vi "CRYCurve Library Socket.vi"(10 "sDataIn":string, 11 "sAction":string) -> (3 "sDataOut":string)   [LabVIEW 2013]
uses:
  Control/CRYCurve Library Cluster.ctl
  CRYSystem/Typedef Control/CRYData Cluster Array.ctl
  CRYSystem/Typedef Control/CRYData Cluster.ctl
  CRYSystem/Typedef Control/CRYResult Cluster Array.ctl
  CRYSystem/Typedef Control/CRYResult Cluster.ctl
  CRYSystem/Typedef Control/CRYWaveform Cluster Array.ctl
  CRYSystem/Typedef Control/CRYWaveform Cluster.ctl
  Global/CRYCurve Library Global.vi
  CRYProject/CRYProject Editor Global.vi
panel:
  in  "CurLib Cluster":T1 {"Waveforms"."Y dB ref" format="%.1f"; "Waveforms"."Y axis" items=["Log", "Lin"]; "Waveforms"."Y data" items=["dB", "Lin"]; "Waveforms"."X data" items=["dB", "Lin"]; "Values"."Z data" items=["dB", "Lin"]; "Values"."X data" items=["dB", "Lin"]; "Values"."Y data" items=["dB", "Lin"]; "Values"."Z dB ref" format="%.1f"; "Values"."Z axis" items=["Log", "Lin"]; "Values"."X dB ref" format="%.1f"; "Values"."X axis" items=["Log", "Lin"]; "Values"."Y axis" items=["Log", "Lin"]; "Values"."Y dB ref" format="%.1f"; "Values"."Curve"."z" format="%.2f"; "Values"."Curve"."y" format="%.2f"; "Values"."Curve"."x" format="%.2f"; "Results"."Margin" format="%.2f"; "Curves"."Z data" items=["dB", "Lin"]; "Curves"."X data" items=["dB", "Lin"]; "Curves"."Y data" items=["dB", "Lin"]; "Curves"."Z dB ref" format="%.1f"; "Curves"."Z axis" items=["Log", "Lin"]; "Curves"."X dB ref" format="%.1f"; "Curves"."X axis" items=["Log", "Lin"]; "Curves"."Y axis" items=["Log", "Lin"]; "Curves"."Y dB ref" format="%.1f"; "Curves"."Curve"."z" format="%.2f"; "Curves"."Curve"."y" format="%.2f"; "Curves"."Curve"."x" format="%.2f"}
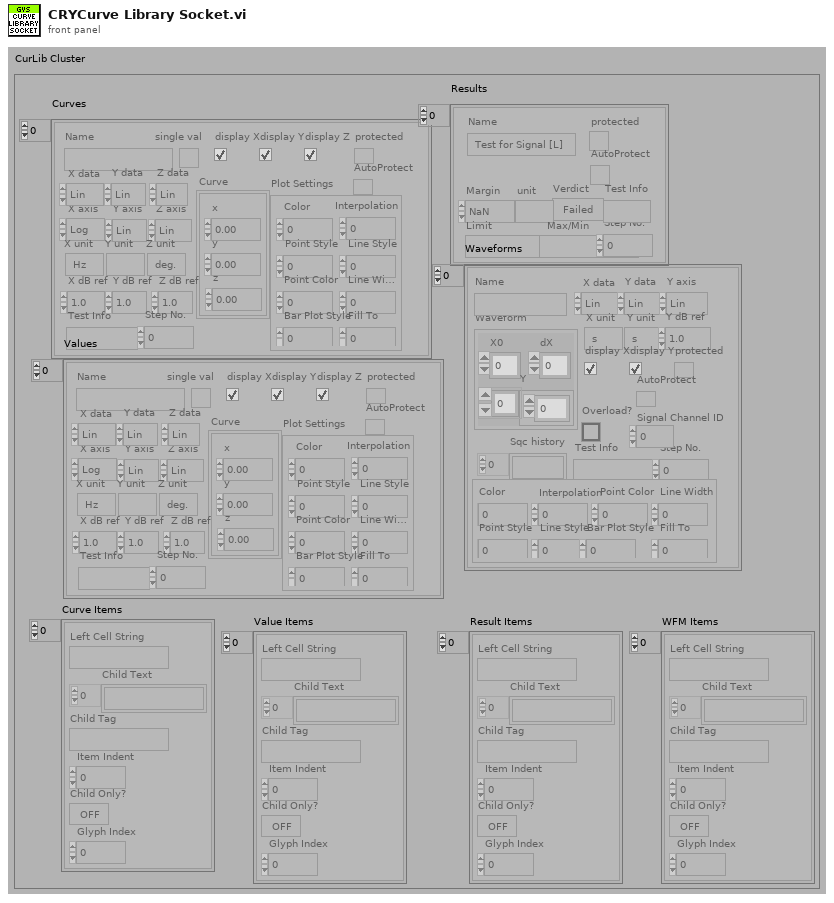
[diagram p1: front panel]
types:
  T1 = typedef "CRYCurve Library Cluster.ctl" = cluster{"Curves":T2, "Results":T4, "Values":T2, "Waveforms":T6, "Curve Items":cluster{"Left Cell String":string, "Child Text":string[], "Child Tag":string, "Item Indent":i32, "Child Only?":bool, "Glyph Index":i32}[], "Value Items":cluster{"Left Cell String":string, "Child Text":string[], "Child Tag":string, "Item Indent":i32, "Child Only?":bool, "Glyph Index":i32}[], "Result Items":cluster{"Left Cell String":string, "Child Text":string[], "Child Tag":string, "Item Indent":i32, "Child Only?":bool, "Glyph Index":i32}[], "WFM Items":cluster{"Left Cell String":string, "Child Text":string[], "Child Tag":string, "Item Indent":i32, "Child Only?":bool, "Glyph Index":i32}[]}
  T2 = typedef "CRYData Cluster Array.ctl" = T3[]
  T3 = typedef "CRYData Cluster.ctl" = cluster{"Name":string, "Curve":cluster{"x":dbl, "y":dbl, "z":dbl}[], "X data":u16, "Y data":u16, "Z data":u16, "X axis":u16, "Y axis":u16, "Z axis":u16, "X unit":string, "Y unit":string, "Z unit":string, "X dB ref":dbl, "Y dB ref":dbl, "Z dB ref":dbl, "single val":bool, "protected":bool, "display X":bool, "display Y":bool, "display Z":bool, "Test Info":string, "Step No.":i32, "Plot Settings":cluster{"Color":u32, "Interpolation":u8, "Point Style":u8, "Line Style":u8, "Point Color":u32, "Line Width":u8, "Bar Plot Style":u8, "Fill To":i16}, "AutoProtect":bool}
  T4 = typedef "CRYResult Cluster Array.ctl" = T5[]
  T5 = typedef "CRYResult Cluster.ctl" = cluster{"Name":string, "Margin":dbl, "unit":string, "Verdict":bool, "Limit":string, "Max/Min":string, "protected":bool, "Step No.":i32, "Test Info":string, "AutoProtect":bool}
  T6 = typedef "CRYWaveform Cluster Array.ctl" = T7[]
  T7 = typedef "CRYWaveform Cluster.ctl" = cluster{"Waveform":cluster{"X0":dbl, "dX":dbl, "Y":sgl[]}, "X data":u16, "Y data":u16, "Y axis":u16, "X unit":string, "Y unit":string, "Y dB ref":dbl, "display Y":bool, "display X":bool, "Overload?":bool, "Test Info":string, "Step No.":i32, "Name":string, "protected":bool, "Sqc history":string[], "Signal Channel ID":i32, "Plot Settings":cluster{"Color":u32, "Interpolation":u8, "Point Style":u8, "Line Style":u8, "Point Color":u32, "Line Width":u8, "Bar Plot Style":u8, "Fill To":i16}, "AutoProtect":bool}
  T8 = cluster{"Left Cell String":string, "Child Text":string[], "Child Tag":string, "Item Indent":i32, "Child Only?":bool, "Glyph Index":i32}[]
  T9 = typedef "CRYCurveLib Info Cluster.ctl" = cluster{"GroupingState":string}
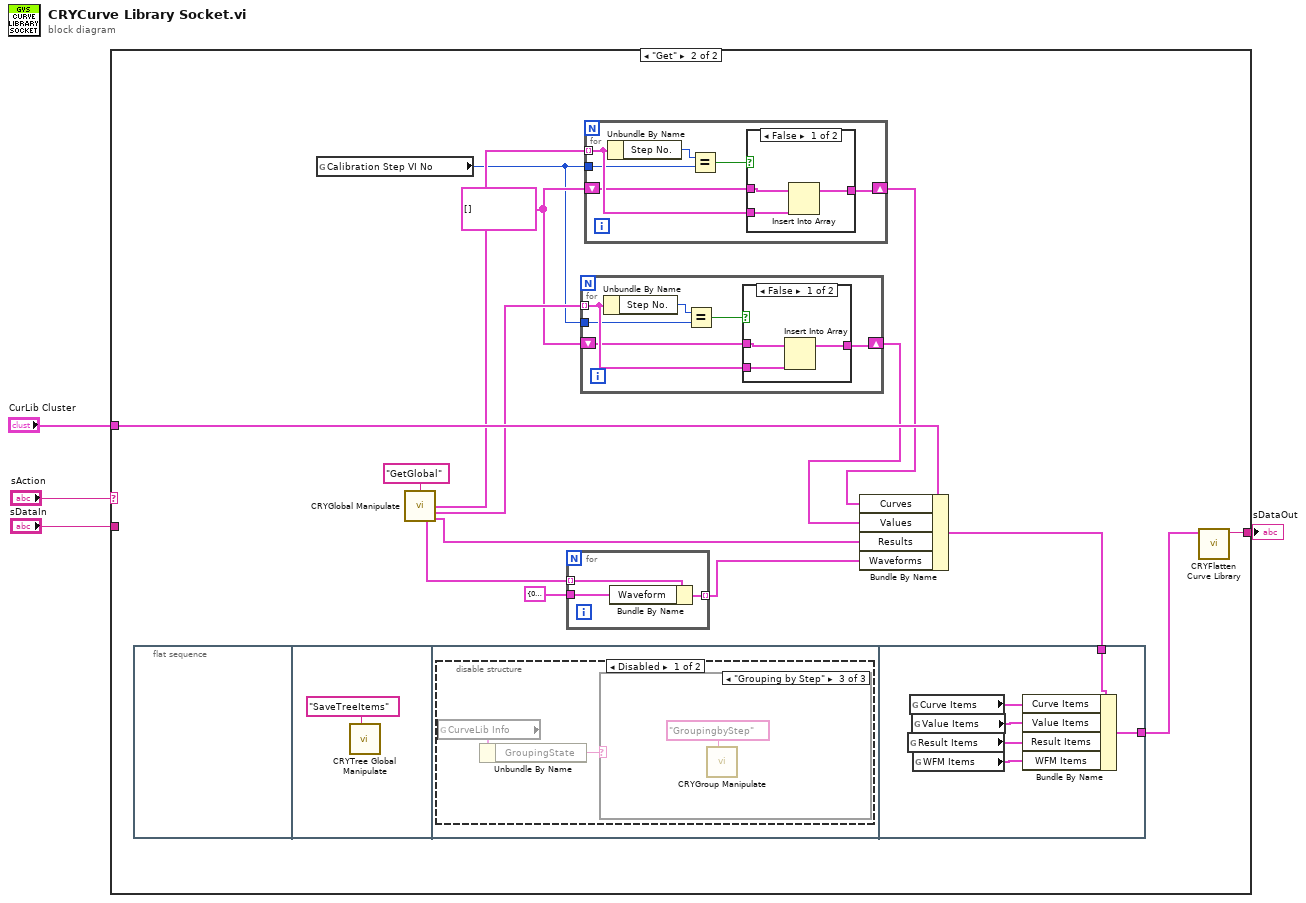
[diagram p0: block diagram]
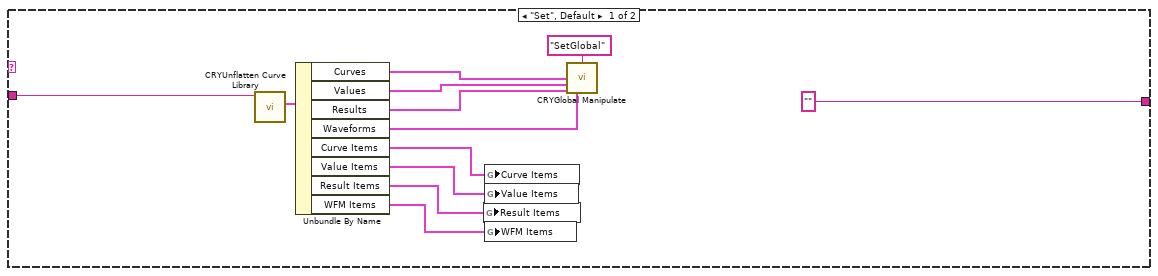
[diagram p2: hidden frame]
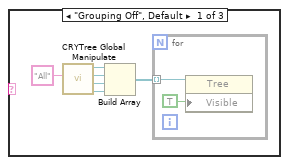
[diagram p5: hidden frame]
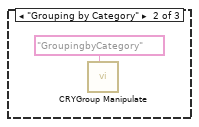
[diagram p6: hidden frame]
diagram:
  n1 = case shown="\"Get\"" "sAction" {
    tunnel: "CurLib Cluster" -> [_ w31]
    tunnel: ["" ("CurLib flattened") w30] -> w2
    tunnel: "sDataIn" -> [w15 _]
    frame "Set", Default {
      n2 = call "CRYUnflatten Curve Library.vi"("Flatten CurLib"=w15) -> ("CurLib Cluster"=w14:T1)  [unwired: 8 in, 2 out]
      n3 = Unbundle By Name(w14) -> ("Curves"=w12:T2, "Values"=w11:T2, "Results"=w9:T4, "Waveforms"=w10:T6, "Curve Items"=w8:T8, "Value Items"=w7:T8, "Result Items"=w6:T8, "WFM Items"=w5:T8)
      n4 = global write "CRYCurve Library Global.vi" "Result Items"(w6) -> ()
      n5 = global write "CRYCurve Library Global.vi" "Curve Items"(w8) -> ()
      n6 = global write "CRYCurve Library Global.vi" "Value Items"(w7) -> ()
      n7 = global write "CRYCurve Library Global.vi" "WFM Items"(w5) -> ()
      n8 = call "CRYGlobal Manipulate.vi"("sAction"="SetGlobal", "Curves"=w12, "Values"=w11, "Results"=w9, "WFM"=w10) -> ()  [unwired: 4 in, 7 out]
    }
    frame "Get" {
      w18 = T2 [] ("Curves")
      n9 = flat-sequence {
        tunnel: w24 -> [w70]
        tunnel: [w69] -> w23
        frame #0 {
        }
        frame #1 {
          n10 = call "CRYTree Global Manipulate.vi"("sAction"="SaveTreeItems") -> ()  [unwired: 7 in, 4 out]
        }
        frame #2 {
          n11 = disable-structure shown="Disabled" {
            frame Disabled {
              n12 = global read "CRYCurve Library Global.vi" "CurveLib Info"() -> (w53:T9)
              n13 = Unbundle By Name(w53) -> ("GroupingState"=w54:string)
              n14 = case shown="\"Grouping by Step\"" w54 {
                frame "Grouping Off", Default {
                  n15 = call "CRYTree Global Manipulate.vi"("sOption"="All") -> ("WFM Tree"=w56:refnum<vi>, "Results Tree"=w57:refnum<vi>, "Values Tree"=w58:refnum<vi>, "Tree/Curve Tree"=w59:refnum<vi>)  [unwired: 7 in]
                  n16 = Build Array(w59, w58, w57, w56) -> (w55:refnum<vi>[])
                  n17 = for {
                    tunnel: w55 -> [w62] mode=indexing
                    n18 = property class="Tree"(reference=w62, "Visible"=TRUE) -> ()  [unwired: 1 in, 2 out]
                  }
                }
                frame "Grouping by Category" {
                  n19 = call "CRYGroup Manipulate.vi"("sAction"="GroupingbyCategory") -> ()  [unwired: 7 in, 4 out]
                }
                frame "Grouping by Step" {
                  n20 = call "CRYGroup Manipulate.vi"("sAction"="GroupingbyStep") -> ()  [unwired: 7 in, 4 out]
                }
              }
            }
            frame Enabled {
            }
          }
        }
        frame #3 {
          n21 = global read "CRYCurve Library Global.vi" "Result Items"() -> (w66:T8)
          n22 = global read "CRYCurve Library Global.vi" "Curve Items"() -> (w68:T8)
          n23 = global read "CRYCurve Library Global.vi" "Value Items"() -> (w67:T8)
          n24 = global read "CRYCurve Library Global.vi" "WFM Items"() -> (w65:T8)
          n25 = Bundle By Name(cluster=w70, "Curve Items"=w68, "Value Items"=w67, "Result Items"=w66, "WFM Items"=w65) -> (w69:T1)
        }
      }
      n26 = global read "CRYProject Editor Global.vi" "Calibration Step VI No"() -> (w17:i32)
      n27 = call "CRYGlobal Manipulate.vi"("sAction"="GetGlobal") -> ("Curves Out"=w22:T3[], "Values Out"=w20:T3[], "WFM Out"=w25:T7[], "Results Out"=w26:T5[])  [unwired: 8 in, 3 out]
      n28 = for {
        tunnel: w25 -> [w73] mode=indexing
        tunnel: cluster{"X0":dbl, "dX":dbl, "Y":sgl[]} {"X0"=0.0, "dX"=0.0, "Y"=[]} ("Waveform") -> [w72]
        tunnel: [w71] -> w28 mode=indexing
        n29 = Bundle By Name(cluster=w73, "Waveform"=w72) -> (w71:T7)
      }
      n30 = for {
        tunnel: w20 -> [w36] mode=indexing
        shift-right: [w33] -> w19
        shift-left: w18 -> [w34]
        tunnel: w17 -> [w32]
        n31 = Unbundle By Name(w36) -> ("Step No."=w37:i32)
        n32 = Equal?(x=w37, y=w32) -> (x = y?=w35:bool)
        n33 = case shown="False" w35 {
          tunnel: w36 -> [w38 _]
          tunnel: w34 -> [w40 w41]
          tunnel: [w39 w41] -> w33
          frame False {
            n34 = Insert Into Array(array=w40, new element=w38) -> (w39:T2)  [unwired: 1 in]
          }
          frame True {
          }
        }
      }
      n35 = for {
        tunnel: w22 -> [w46] mode=indexing
        shift-right: [w43] -> w21
        shift-left: w18 -> [w44]
        tunnel: w17 -> [w42]
        n36 = Unbundle By Name(w46) -> ("Step No."=w47:i32)
        n37 = Equal?(x=w47, y=w42) -> (x = y?=w45:bool)
        n38 = case shown="False" w45 {
          tunnel: w46 -> [w48 _]
          tunnel: w44 -> [w50 w51]
          tunnel: [w49 w51] -> w43
          frame False {
            n39 = Insert Into Array(array=w50, new element=w48) -> (w49:T2)  [unwired: 1 in]
          }
          frame True {
          }
        }
      }
      n40 = Bundle By Name(cluster=w31, "Curves"=w21, "Values"=w19, "Results"=w26, "Waveforms"=w28) -> (w24:T1)
      n41 = call "CRYFlatten Curve Library.vi"("CurLibData"=w23) -> ("CurLib flattened"=w30:string)  [unwired: 10 in]
    }
  }
  "sDataOut" <- w2
